vi "DeviceReset.vi"(9 "Reserved":u32, 10 "DeviceInd":u32, 11 "DeviceType":u32) -> (3 "Success":bool)   [LabVIEW 2011]
uses:
  data/ControlCAN.dll
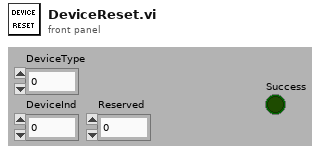
[diagram p1: front panel]
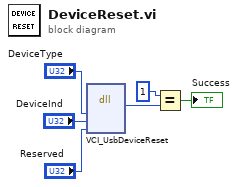
[diagram p0: block diagram]
diagram:
  n1 = dll-call lib="PTH1Nabs D\t董海成\t上位机2.进行中USB-CAN TooldataControlCAN.dll" fn="VCI_UsbDeviceReset" ("VCI_FindUsbDevice")("DeviceType"="DeviceType", "DeviceInd"="DeviceInd", "Reserved"="Reserved") -> ("返回类型"=w3:u32)  [unwired: 6 in, 2 out]
  n2 = Equal?(x=u32 1, y=w3) -> (x = y?=→"Success":bool)
